vi "PXF4_get_hysteresis.vi"(8 "error in":errorcluster, 11 "Modbus Master in":refnum<class "Modbus Master.lvclass">) -> (0 "error out":errorcluster, 2 "hysteresis":i16, 3 "Modbus Master out":refnum<class "Modbus Master.lvclass">)   [LabVIEW 2019]
uses:
  <vilib>/NI/Modbus Library/API/Master/Modbus Master.lvclass
panel:
  out "hysteresis_raw":u16
  out "register values":u16[](array[numeric])
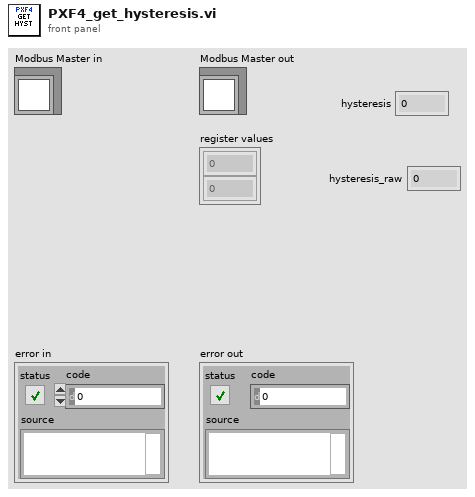
[diagram p1: front panel]
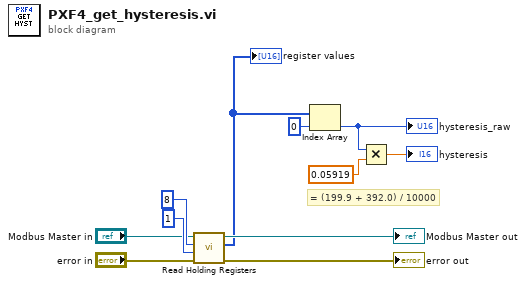
[diagram p0: block diagram]
diagram:
  # "= (199.9 + 392.0) / 10000"
  n1 = call-dynamic "Read Holding Registers.vi"("error in"="error in", "number of inputs"=u16 1, "starting address"=u16 8, "Modbus master in"="Modbus Master in") -> ("error out"=→"error out":errorcluster, "register values"=w5:u16[], "Modbus master out"=→"Modbus Master out":refnum<class "Modbus Master.lvclass">)  [unwired: 5 in]
  "register values" <- w5
  n2 = Index Array(array=w5, index=0) -> (element=w2:u16)
  "hysteresis_raw" <- w2
  n3 = Multiply(x=w2, y=0.05919) -> (x*y=→"hysteresis":dbl)
